vi "setChannels_inUse.vi"(8 "error in (no error)":errorcluster, 10 "channels_inUse":T1(array[cluster]), 11 "device.lvclass in":refnum<class "device.lvclass">) -> (0 "error out":errorcluster, 3 "device.lvclass out":refnum<class "device.lvclass">)   [LabVIEW 2011, in "Tools.lvlib" / "DatabaseHelpers.lvlib" / "device.lvclass"]
uses:
  device.lvclass
  device.lvclass/device.ctl
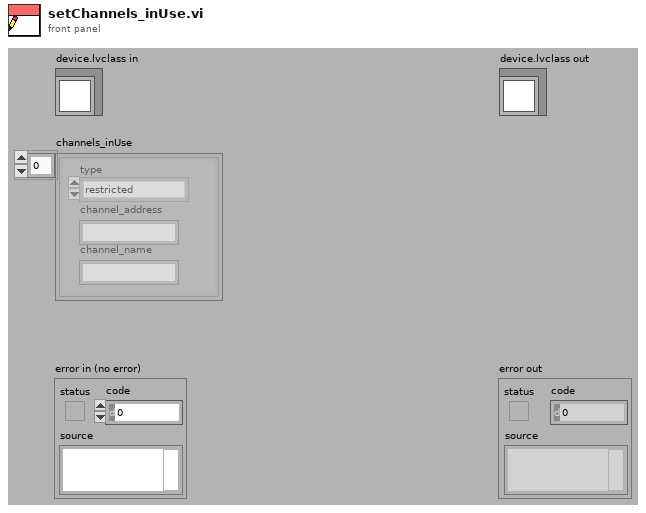
[diagram p1: front panel]
types:
  T1 = cluster{"type":enum16{"restricted", "unrestricted"}, "channel_address":string, "channel_name":string}[]
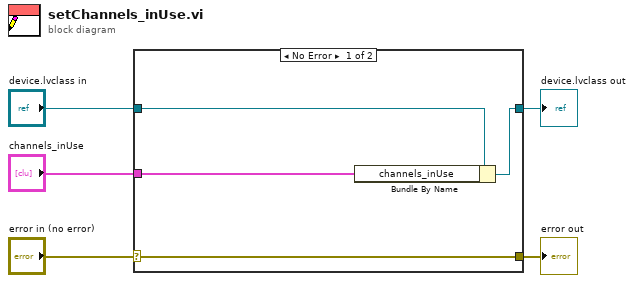
[diagram p0: block diagram]
diagram:
  n1 = case shown="No Error" "error in (no error)" {
    selector: "error in (no error)" -> [w9 w10]
    tunnel: [w9 w10] -> w4
    tunnel: [w7 w11] -> w2
    tunnel: "device.lvclass in" -> [w8 w11]
    tunnel: "channels_inUse" -> [w6 _]
    frame No Error {
      n2 = Bundle By Name(cluster=w8, "channels_inUse"=w6) -> (w7:refnum<class "device.lvclass">)
    }
    frame Error {
    }
  }
  "error out" <- w4
  "device.lvclass out" <- w2
